vi "X_Limit_Length_Value_Change.vi"(1 "Max String Length":i32, 2 "Char":i16, 3 "Input String":string) -> (0 "Result String":string)   [LabVIEW 2012, in "String_XControl.xctl"]
doc: "This code takes in the last char pressed, the maximum string length, and the current string. The output is a string that is less than or equal to the maximum length."
uses:
  String_XControl.xctl
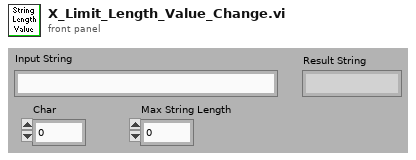
[diagram p1: front panel]
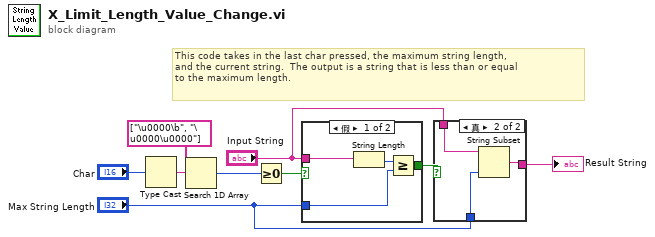
[diagram p0: block diagram]
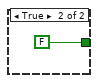
[diagram p3: hidden frame]
diagram:
  # "This code takes in the last char pressed, the maximum string length,\nand the current string.  The output is a string that is less than or equal\nto the maximum length."
  n1 = Type Cast(x="Char") -> (*(type *) &x=w9:string)  [unwired: 1 out]
  n2 = Search 1D Array(1D array=string[] ["\u0000\b", "\u0000\u0000"], element=w9) -> (index of element=w6:i32)  [unwired: 1 out]
  n3 = Greater Or Equal To 0?(x=w6) -> (x >= 0?=w7:bool)
  n4 = case shown="假" w7 {
    tunnel: [w12 FALSE] -> w4
    tunnel: "Max String Length" -> [w11 _]
    tunnel: "Input String" -> [w10 _]
    frame False {
      n5 = String Length(string=w10) -> (length=w13:i32)
      n6 = Greater Or Equal?(x=w13, y=w11) -> (x >= y?=w12:bool)
    }
    frame True {
    }
  }
  n7 = case shown="真" w4 {
    tunnel: [w15 w16] -> w1
    tunnel: "Input String" -> [w15 w18]
    tunnel: "Max String Length" -> [_ w17]
    frame False {
    }
    frame True {
      n8 = String Subset(string=w18, length (rest)=w17) -> (substring=w16:string)  [unwired: 1 out]
    }
  }
  "Result String" <- w1
